vi "Forward Tell.vi"(8 "Error in":errorcluster, 10 "Msg DVR":refnum<data-value>, 11 "TEMPLATE Actor in":refnum<class "{{Name}}Actor.lvclass">) -> (0 "Error out":errorcluster, 3 "TEMPLATE Actor out":refnum<class "{{Name}}Actor.lvclass">)   [LabVIEW 2020, in "_Template.lvlib" / "Templates.lvlib" / "{{Name}}Actor.lvlib" / "{{Name}}Actor.lvclass"]
uses:
  {{Name}}Actor.lvclass
  {{Name}}Actor.lvclass/{{Name}}Actor.ctl
  jettl/jettl/Message.ctl
  jettl/jettl/jettl.lvlib
  jettl/jettl/Message/Message.lvclass
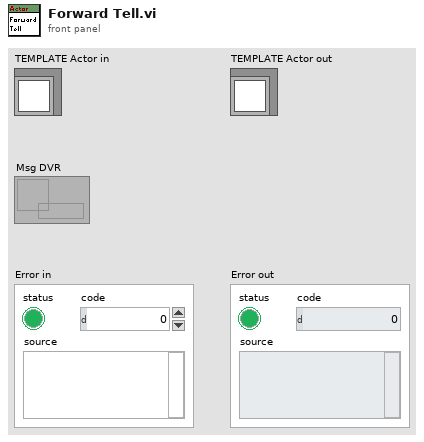
[diagram p1: front panel]
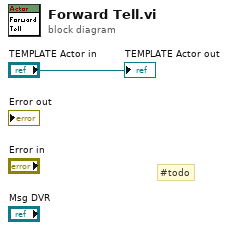
[diagram p0: block diagram]
diagram:
  # "#todo"
  "TEMPLATE Actor out" <- "TEMPLATE Actor in"
